vi "AMC Three Button Dialog.vi"(4 "Allow user to close window? (TRUE)":bool=TRUE, 5 "Justify Message (Left)":enum16{"Left", "Center", "Right"}(ring), 6 "Keyboard Shortcuts (Left is <Enter>)":T2={"Left Button Key Shortcut"={"Control"=FALSE, "Shift"=FALSE, "Key"="<Enter>"}, "Center Button Key Shortcut"={"Control"=FALSE, "Shift"=FALSE, "Key"=""}, "Right Button Key Shortcut"={"Control"=FALSE, "Shift"=FALSE, "Key"=""}}, 7 "Window Title (\"\")":string, 8 "Right Button Text (\"Cancel\")":string="Cancel", 9 "Center Button Text (\"No\")":string="No", 10 "Left Button Text (\"Yes\")":string="Yes", 11 "message":string) -> (3 "Which Button?":T3(ring)=enum."Center Button")   [LabVIEW 2009]
doc: "Displays text in a dialog with three buttons. The output enum indicates which of the three buttons the user chose, or it indicates that the user closed the dialog without making any choice."
uses:
  vi.lib/NI/AMC/AMC.lvlib
panel:
  in  "State Variables":T1={"Justify Message"=enum."Left", "message"="", "Left Button Text"="Yes", "Center Button Text"="No", "Right Button Text"="Cancel", "Keyboard Shortcuts"={"Left Button Key Shortcut"={"Control"=FALSE, "Shift"=FALSE, "Key"="<Enter>"}, "Center Button Key Shortcut"={"Control"=FALSE, "Shift"=FALSE, "Key"=""}, "Right Button Key Shortcut"={"Control"=FALSE, "Shift"=FALSE, "Key"=""}}, "Left Button Visible"=FALSE, "Center Button Visible"=FALSE, "Right Button Visible"=FALSE, "Minimum window width for buttons"=0, "Mimimum window width"=0, "Minimum width for message"=0, "FP Spacing"=12, "Height"=0, "Actual Width"=0, "Left Edge"=0, "FP Window Title"=""}
  in  "OK":string="OK"
  out "C-Message":string
  in  "Right Button":bool
  in  "Center Button":bool
  in  "Left Button":bool
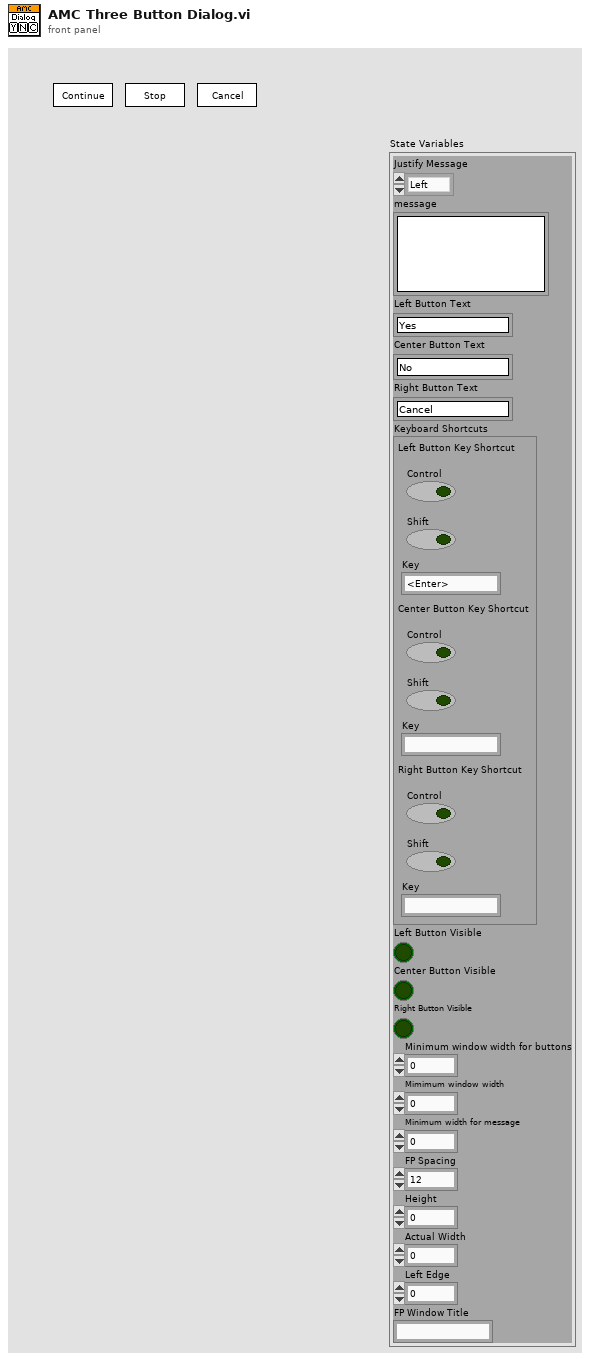
[diagram p1: front panel]
types:
  T1 = cluster{"Justify Message":enum16{"Left", "Center", "Right"}, "message":string, "Left Button Text":string, "Center Button Text":string, "Right Button Text":string, "Keyboard Shortcuts":cluster{"Left Button Key Shortcut":cluster{"Control":bool, "Shift":bool, "Key":string}, "Center Button Key Shortcut":cluster{"Control":bool, "Shift":bool, "Key":string}, "Right Button Key Shortcut":cluster{"Control":bool, "Shift":bool, "Key":string}}, "Left Button Visible":bool, "Center Button Visible":bool, "Right Button Visible":bool, "Minimum window width for buttons":i32, "Mimimum window width":i32, "Minimum width for message":i32, "FP Spacing":i32, "Height":u32, "Actual Width":i32, "Left Edge":i32, "FP Window Title":string}
  T2 = cluster{"Left Button Key Shortcut":cluster{"Control":bool, "Shift":bool, "Key":string}, "Center Button Key Shortcut":cluster{"Control":bool, "Shift":bool, "Key":string}, "Right Button Key Shortcut":cluster{"Control":bool, "Shift":bool, "Key":string}}
  T3 = enum16{"Left Button", "Center Button", "Right Button", "Window Close"}
  T4 = typedef "AMC.lvlib/Message Queue.ctl" = refnum<queue>
  T5 = cluster{"left":i16, "top":i16, "right":i16, "bottom":i16}
  T6 = cluster{"Control":bool, "Shift":bool, "Key":string}
  T7 = cluster{bool, "Control":bool, "Shift":bool, "Key":string}
  T8 = typedef "LVRectTypeDef.ctl" = cluster{"left":i16, "top":i16, "right":i16, "bottom":i16}
  T9 = typedef "LVPointTypeDef.ctl" = cluster{"Horizontal":i16, "Vertical":i16}
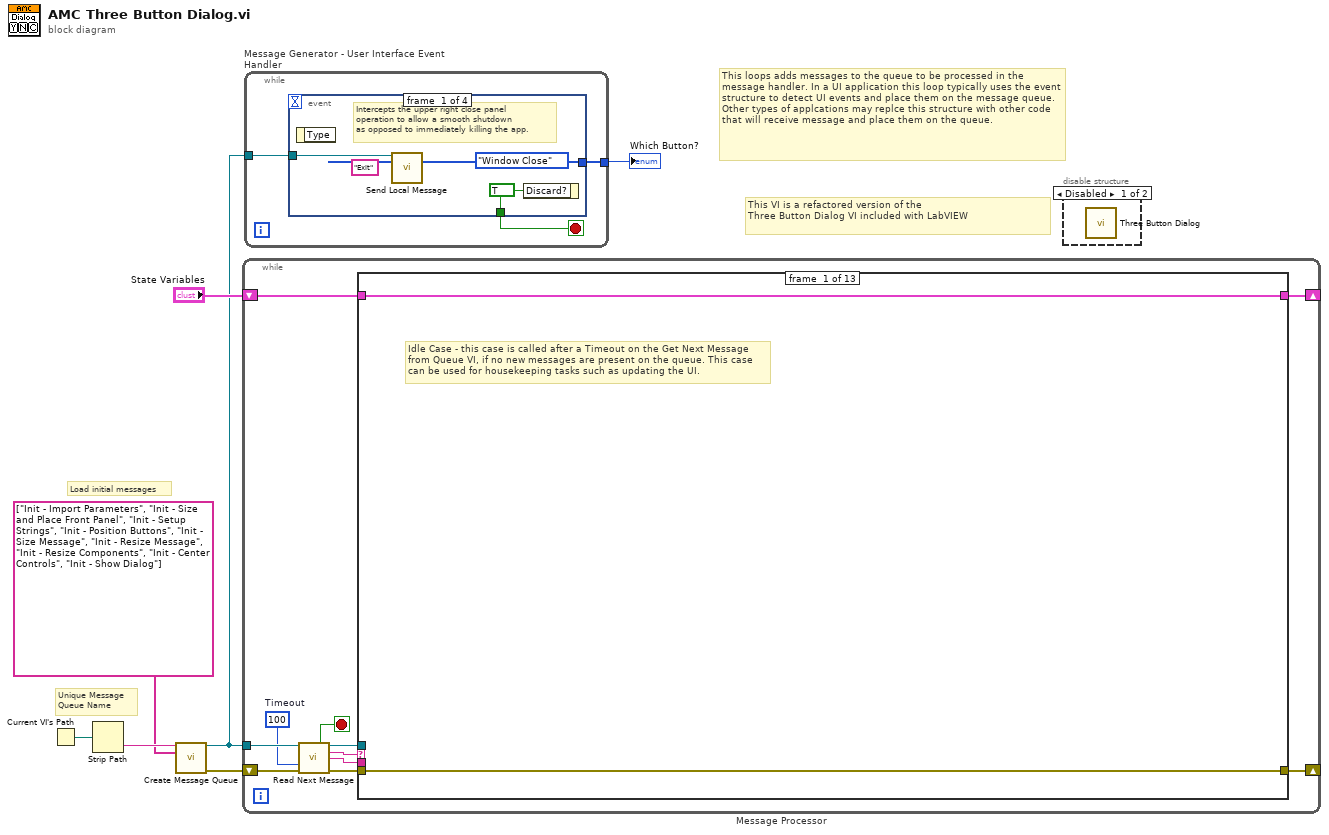
[diagram p0: block diagram]
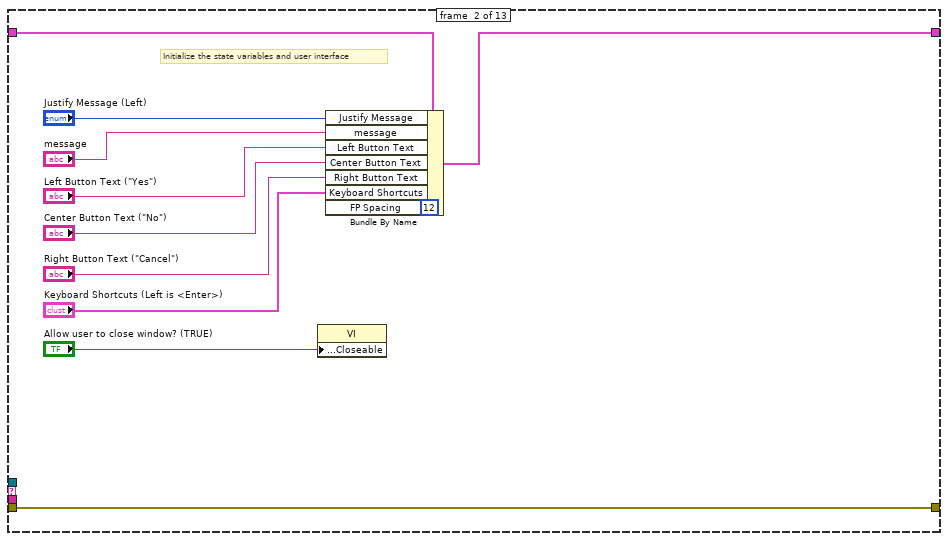
[diagram p3: hidden frame]
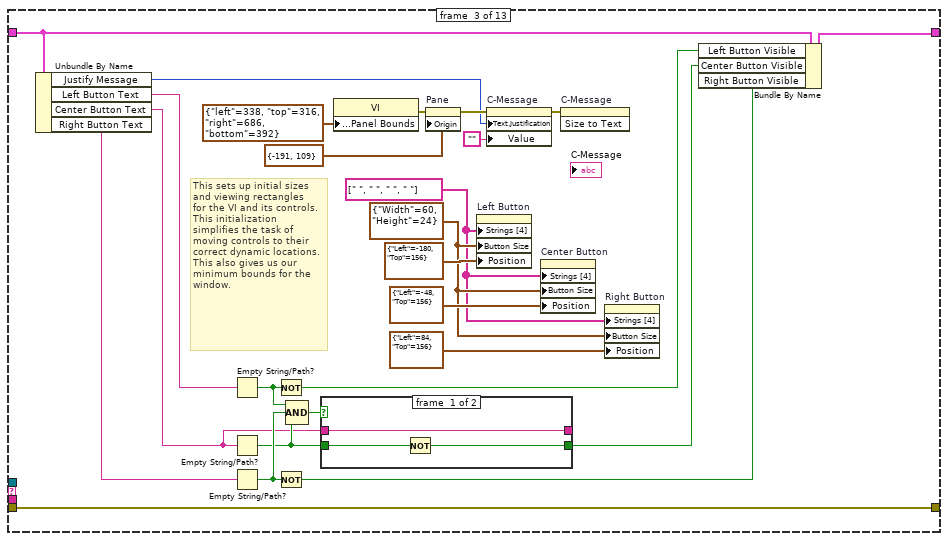
[diagram p4: hidden frame]
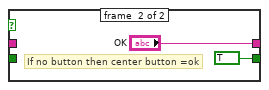
[diagram p5: hidden frame]
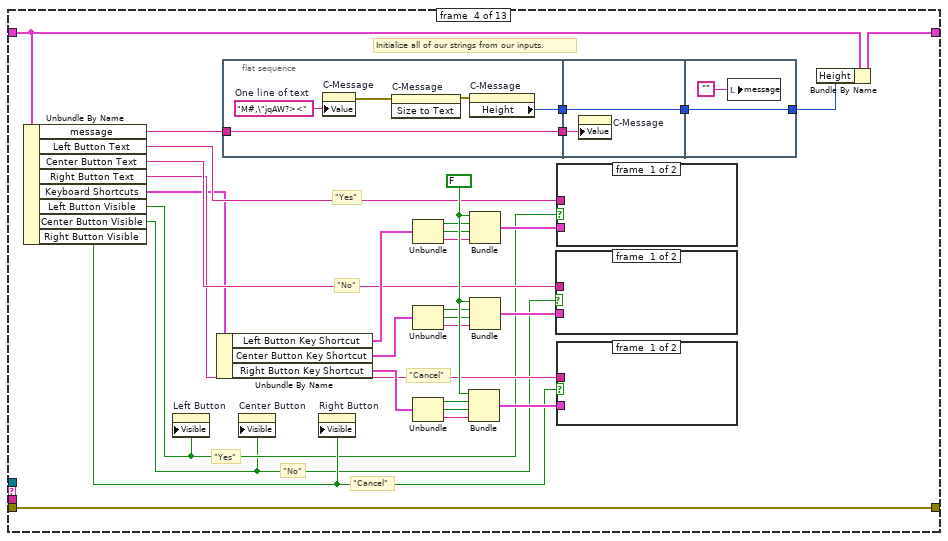
[diagram p6: hidden frame]
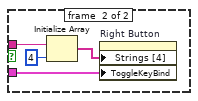
[diagram p7: hidden frame]
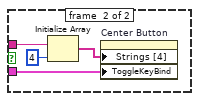
[diagram p8: hidden frame]
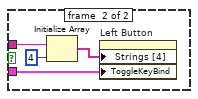
[diagram p9: hidden frame]
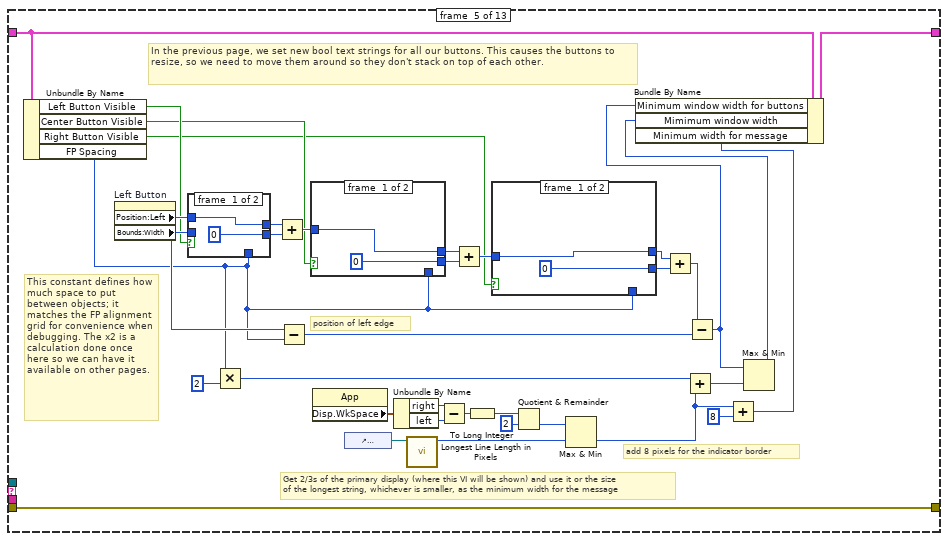
[diagram p10: hidden frame]
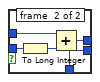
[diagram p11: hidden frame]
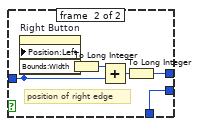
[diagram p12: hidden frame]
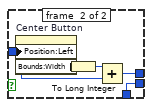
[diagram p13: hidden frame]
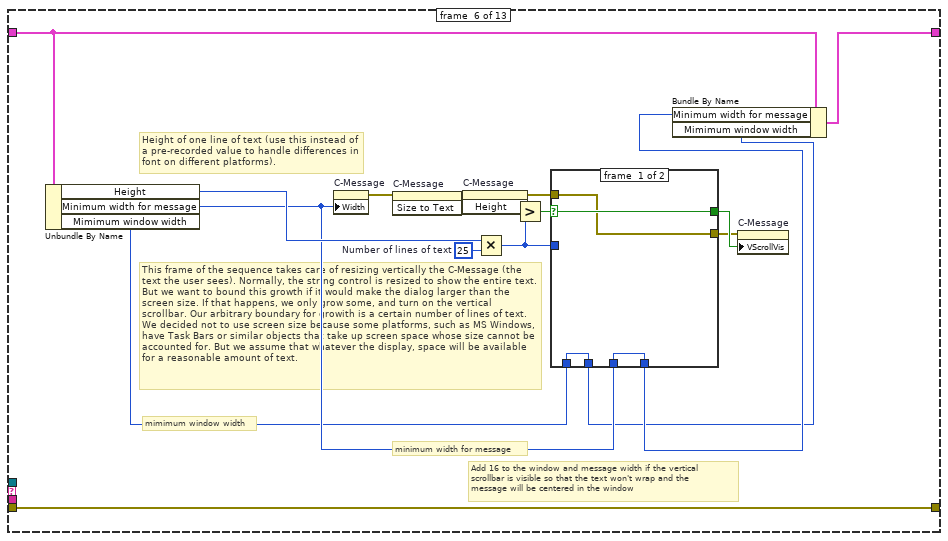
[diagram p14: hidden frame]
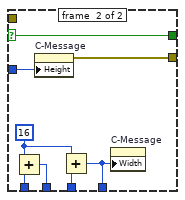
[diagram p15: hidden frame]
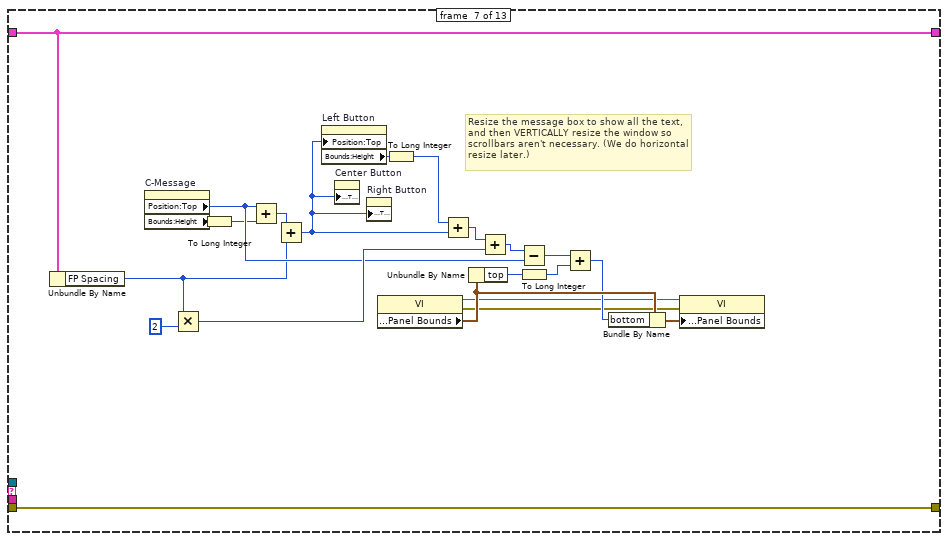
[diagram p16: hidden frame]
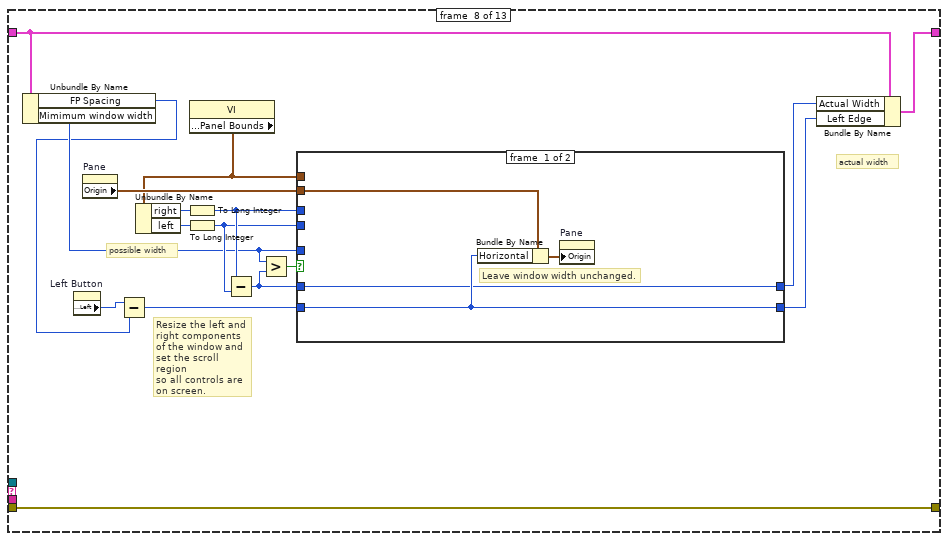
[diagram p17: hidden frame]
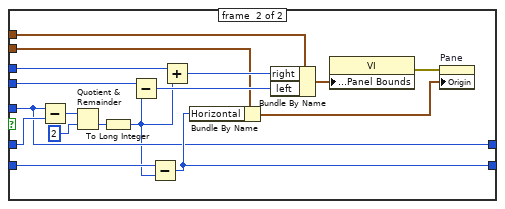
[diagram p18: hidden frame]
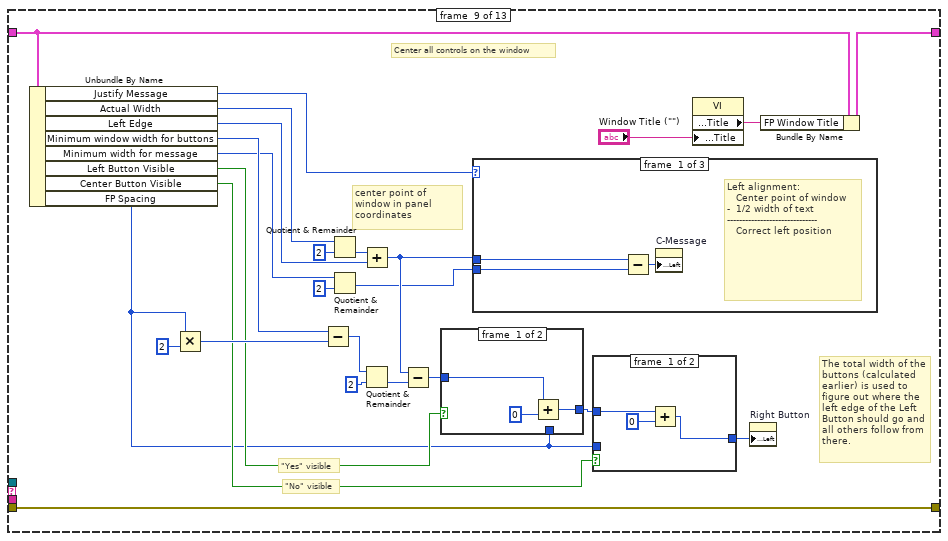
[diagram p19: hidden frame]
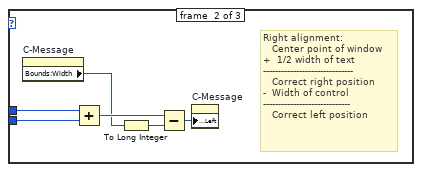
[diagram p20: hidden frame]
diagram:
  # "This VI is a refactored version of the\nThree Button Dialog VI included\twith LabVIEW"
  # "This loops adds messages to the queue to be processed in the message handler. In a UI application this loop typically uses the event structure to detect UI events and place them on the message queue. Other types of applcations may replce this structure with other code that will receive message and place them on the queue."
  # "Unique Message\nQueue Name"
  # "Load initial messages"
  n1 = Current VI's Path() -> (path=w6:path)
  n2 = Strip Path(path=w6) -> (name=w7:string)  [unwired: 1 out]
  n3 = call "Create Message Queue.vi"("message queue name"=w7, "initial message names"=string[] ["Init - Import Parameters", "Init - Size and Place Front Panel", "Init - Setup Strings", "Init - Position Buttons", "Init - Size Message", "Init - Resize Message", "Init - Resize Components", "Init - Center Controls", "Init - Show Dialog"]) -> ("message queue out"=w4:T4, "error out"=w3:errorcluster)  [unwired: 12 in]
  n4 = while "Message Processor" {
    shift-left: w3 -> [w12]
    shift-right: [w13] -> _
    tunnel: w4 -> [w11]
    shift-left: "State Variables" -> [w18]
    shift-right: [w17] -> _
    stop <- w16 stop-if-true
    w8 = 100  # Timeout
    n5 = call "Read Next Message.vi"("message queue in"=w11, "timeout (1 ms)"=w8, "error in"=w12) -> ("exit process?"=w16:bool, "message queue out"=w15:T4, "message name"=w10:string, "message value"=w9:string, "error out"=w14:errorcluster)  [unwired: 5 in, 3 out]
    n6 = case shown="\"Error\"" w10 {
      selector: w10 -> [_ _ _ _ _ _ _ _ _ _ _ _ w343]
      tunnel: [w20 w30 w37 w64 w149 w175 w203 w225 w283 w321 w334 w336 w345] -> w17
      tunnel: w18 -> [w20 w31 w38 w65 w122 w176 w203 w229 w285 w321 w334 w336 w345]
      tunnel: w15 -> [_ _ _ _ _ _ _ _ _ _ w332 w339 _]
      tunnel: w14 -> [w19 w22 w32 w62 w114 w172 w201 w224 w262 w323 _ w340 w344]
      tunnel: [w19 w22 w32 w62 w114 w172 w201 w224 w262 w323 errorcluster {"status"=FALSE, "code"=0, "source"=""} ("error out") w338 w344] -> w13
      tunnel: w9 -> [_ _ _ _ _ _ _ _ _ _ _ _ _]
      frame #0 {
        # "Idle Case - this case is called after a Timeout on the Get Next Message from Queue VI, if no new messages are present on the queue. This case can be used for housekeeping tasks such as updating the UI."
      }
      frame #1 {
        # "Initialize the state variables and user interface"
        n7 = property class="VI"("Front Panel Window:Closeable"="Allow user to close window? (TRUE)") -> ()  [unwired: 2 in, 2 out]
        n8 = Bundle By Name(cluster=w31, "Justify Message"="Justify Message (Left)", "message"="message", "Left Button Text"="Left Button Text (\"Yes\")", "Center Button Text"="Center Button Text (\"No\")", "Right Button Text"="Right Button Text (\"Cancel\")", "Keyboard Shortcuts"="Keyboard Shortcuts (Left is <Enter>)", "FP Spacing"=12) -> (w30:T1)
      }
      frame #2 {
        w46 = string[] [" ", " ", " ", " "] ("Strings [4]")
        w47 = cluster{"Width":u32, "Height":u32} {"Width"=60, "Height"=24} ("Button Size")
        # "This sets up initial sizes and viewing rectangles\nfor the VI and its controls. This initialization\nsimplifies the task of moving controls to their\ncorrect dynamic locations. This also gives us our\nminimum bounds for the window."
        n9 = Unbundle By Name(w38) -> ("Justify Message"=w36:enum16{"Left", "Center", "Right"}, "Left Button Text"=w39:string, "Center Button Text"=w40:string, "Right Button Text"=w41:string)
        n10 = Empty String/Path?(string/path=w39) -> (empty?=w42:bool)
        n11 = Empty String/Path?(string/path=w40) -> (empty?=w44:bool)
        n12 = Empty String/Path?(string/path=w41) -> (empty?=w45:bool)
        n13 = Not(x=w42) -> (.not. x?=w33:bool)
        n14 = Not(x=w45) -> (.not. x?=w35:bool)
        n15 = Compound Arithmetic op=AND(w42, w45, w44) -> (w43:bool)
        n16 = case shown="True" w43 {
          tunnel: w44 -> [w59 _]
          tunnel: [w58 TRUE] -> w34
          tunnel: w40 -> [w57 _]
          tunnel: [w57 "OK"] -> _
          frame #0 {
            n17 = Not(x=w59) -> (.not. x?=w58:bool)
          }
          frame #1 {
            # "If no button then center button =ok"
          }
        }
        n18 = property class="VI"("Front Panel Window:Panel Bounds"=T5 {"left"=338, "top"=316, "right"=686, "bottom"=392} ("Front Panel.PanelBounds")) -> (error out=w54:errorcluster)  [unwired: 2 in, 1 out]
        n19 = property on="Pane" class="Pane"(error in=w54, "Origin"=cluster{"Horizontal":i16, "Vertical":i16} {"Horizontal"=-191, "Vertical"=109} ("Front Panel.Origin")) -> (error out=w55:errorcluster)  [unwired: 1 in, 1 out]
        n20 = property on="Left Button" class="Boolean"("Strings [4]"=w46, "Button Size"=w47, "Position"=cluster{"Left":i32, "Top":i32} {"Left"=-180, "Top"=156}) -> ()  [unwired: 2 in, 2 out]
        n21 = property on="C-Message" class="Str"(error in=w55, "Text.Justification"=w36, "Value"="") -> (error out=w51:errorcluster)  [unwired: 1 in, 1 out]
        n22 = property on="Center Button" class="Bool"("Strings [4]"=w46, "Button Size"=w47, "Position"=cluster{"Left":i32, "Top":i32} {"Left"=-48, "Top"=156}) -> ()  [unwired: 2 in, 2 out]
        n23 = invoke on="C-Message" class="Str" method="Size to Text"(error in=w51) -> ()  [unwired: 2 in, 3 out]
        n24 = property on="Right Button" class="Bool"("Strings [4]"=w46, "Button Size"=w47, "Position"=cluster{"Left":i32, "Top":i32} {"Left"=84, "Top"=156}) -> ()  [unwired: 2 in, 2 out]
        n25 = Bundle By Name(cluster=w38, "Left Button Visible"=w33, "Center Button Visible"=w34, "Right Button Visible"=w35) -> (w37:T1)
      }
      frame #3 {
        w86 = FALSE
        # "\"Cancel\""
        # "\"No\""
        # "\"Yes\""
        # "\"Cancel\""
        # "\"No\""
        # "\"Yes\""
        # "Initialize all of our strings from our inputs."
        n26 = Unbundle By Name(w65) -> ("message"=w89:string, "Left Button Text"=w72:string, "Center Button Text"=w71:string, "Right Button Text"=w70:string, "Keyboard Shortcuts"=w69:T2, "Left Button Visible"=w67:bool, "Center Button Visible"=w66:bool, "Right Button Visible"=w68:bool)
        n27 = property on="Left Button" class="Boolean"("Visible"=w67) -> ()  [unwired: 2 in, 2 out]
        n28 = Unbundle By Name(w69) -> ("Left Button Key Shortcut"=w73:T6, "Center Button Key Shortcut"=w81:T6, "Right Button Key Shortcut"=w87:T6)
        n29 = flat-sequence {
          tunnel: [w106] -> w92
          tunnel: w89 -> [w105]
          tunnel: [w105] -> w91
          tunnel: w92 -> [w111]
          tunnel: [w111] -> w90
          tunnel: w91 -> [w110]
          tunnel: w90 -> [w112]
          tunnel: [w112] -> w63
          frame #0 {
            w109 = "M#,\"jqAW?><"  # One line of text
            n30 = property on="C-Message" class="Str"("Value"=w109) -> (error out=w107:errorcluster)  [unwired: 2 in, 1 out]
            n31 = invoke on="C-Message" class="Str" method="Size to Text"(error in=w107) -> (error out=w108:errorcluster)  [unwired: 2 in, 2 out]
            n32 = property on="C-Message" class="Str"(error in=w108) -> ("Height"=w106:u32)  [unwired: 1 in, 2 out]
          }
          frame #1 {
            n33 = property on="C-Message" class="Str"("Value"=w110) -> ()  [unwired: 2 in, 2 out]
          }
          frame #2 {
            n34 = local write "message"("") -> ()
          }
        }
        n35 = property on="Center Button" class="Bool"("Visible"=w66) -> ()  [unwired: 2 in, 2 out]
        n36 = property on="Right Button" class="Bool"("Visible"=w68) -> ()  [unwired: 2 in, 2 out]
        n37 = Unbundle(w73) -> ("Control"=w74:bool, "Shift"=w75:bool, "Key"=w76:string)
        n38 = Unbundle(w81) -> ("Control"=w78:bool, "Shift"=w79:bool, "Key"=w80:string)
        n39 = Unbundle(w87) -> ("Control"=w83:bool, "Shift"=w84:bool, "Key"=w85:string)
        n40 = Bundle(w86, "Control"=w83, "Shift"=w84, "Key"=w85) -> (w88:T7)  [unwired: 1 out]
        n41 = Bundle(w86, "Control"=w74, "Shift"=w75, "Key"=w76) -> (w77:T7)  [unwired: 1 out]
        n42 = Bundle(w86, "Control"=w78, "Shift"=w79, "Key"=w80) -> (w82:T7)  [unwired: 1 out]
        n43 = case shown="True" w66 {
          tunnel: w82 -> [_ w98]
          tunnel: w71 -> [_ w97]
          frame #0 {
          }
          frame #1 {
            n44 = Initialize Array(w97, 4 ("dimension size")) -> (w100:string[])
            n45 = property on="Center Button" class="Bool"("Strings [4]"=w100, "ToggleKeyBind"=w98) -> ()  [unwired: 2 in, 2 out]
          }
        }
        n46 = case shown="True" w67 {
          tunnel: w72 -> [_ w102]
          tunnel: w77 -> [_ w101]
          frame #0 {
          }
          frame #1 {
            n47 = Initialize Array(w102, 4 ("dimension size")) -> (w104:string[])
            n48 = property on="Left Button" class="Boolean"("Strings [4]"=w104, "ToggleKeyBind"=w101) -> ()  [unwired: 2 in, 2 out]
          }
        }
        n49 = case shown="True" w68 {
          tunnel: w88 -> [_ w94]
          tunnel: w70 -> [_ w93]
          frame #0 {
          }
          frame #1 {
            n50 = Initialize Array(w93, 4 ("dimension size")) -> (w96:string[])
            n51 = property on="Right Button" class="Bool"("Strings [4]"=w96, "ToggleKeyBind"=w94) -> ()  [unwired: 2 in, 2 out]
          }
        }
        n52 = Bundle By Name(cluster=w65, "Height"=w63) -> (w64:T1)
      }
      frame #4 {
        # "add 8 pixels for the indicator border"
        # "Get 2/3s of the primary display (where this VI will be shown) and use it or the size\nof the longest string, whichever is smaller, as the minimum width for the message"
        # "This constant defines how much space to put between objects; it matches the FP alignment grid for convenience when debugging. The x2 is a calculation done once here so we can have it available on other pages."
        # "In the previous page, we set new bool text strings for all our buttons. This causes the buttons to resize, so we need to move them around so they don't stack on top of each other."
        # "position of left edge"
        n53 = Unbundle By Name(w122) -> ("Left Button Visible"=w121:bool, "Center Button Visible"=w120:bool, "Right Button Visible"=w119:bool, "FP Spacing"=w118:i32)
        n54 = property on="Left Button" class="Boolean"() -> ("Position:Left"=w126:i32, "Bounds:Width"=w129:u32)  [unwired: 2 in, 2 out]
        n55 = case shown="True" w121 {
          tunnel: w126 -> [w151 w156]
          tunnel: w129 -> [_ w155]
          tunnel: [w151 w154] -> w132
          tunnel: w118 -> [_ w152]
          tunnel: [0 w152] -> w133
          frame #0 {
          }
          frame #1 {
            n56 = To Long Integer(number=w155) -> (32bit integer=w153:i32)
            n57 = Add(x=w156, y=w153) -> (x+y=w154:i32)
          }
        }
        n58 = Multiply(x=w118, y=2) -> (x*y=w138:i32)
        n59 = Add(x=w132, y=w133) -> (x+y=w128:i32)
        n60 = Subtract(x=w126, y=w118) -> (x-y=w125:i32)
        n61 = case shown="True" w120 {
          tunnel: w128 -> [w166 w171]
          tunnel: [w166 w170] -> w130
          tunnel: [0 w167] -> w134
          tunnel: w118 -> [_ w167]
          frame #0 {
          }
          frame #1 {
            n62 = property on="Center Button" class="Bool"("Position:Left"=w171) -> ("Bounds:Width"=w169:u32)  [unwired: 2 in, 2 out]
            n63 = To Long Integer(number=w169) -> (32bit integer=w168:i32)
            n64 = Add(x=w168, y=w171) -> (x+y=w170:i32)
          }
        }
        n65 = property class="App"() -> ("Disp.WkSpace"=w139:T8)  [unwired: 2 in, 2 out]
        n66 = control-ref of="C-Message"() -> (w136:refnum<vi>)
        n67 = Unbundle By Name(w139) -> ("right"=w143:i16, "left"=w144:i16)
        n68 = call <vilib>:"Longest Line Length in Pixels.vi"("String"=w136) -> ("longest line length"=w142:i32)  [unwired: 1 in, 8 out]
        n69 = Subtract(x=w143, y=w144) -> (x-y=w140:i16)
        n70 = Add(x=w130, y=w134) -> (x+y=w127:i32)
        n71 = To Long Integer(number=w140) -> (32bit integer=w145:i32)
        n72 = case shown="True" w119 {
          tunnel: w127 -> [w158 w164]
          tunnel: [w158 w162] -> w131
          tunnel: [0 w159] -> w135
          tunnel: w118 -> [_ w159]
          frame #0 {
          }
          frame #1 {
            # "position of right edge"
            n73 = property on="Right Button" class="Bool"("Position:Left"=w164) -> ("Bounds:Width"=w161:u32)  [unwired: 2 in, 2 out]
            n74 = To Long Integer(number=w161) -> (32bit integer=w160:i32)
            n75 = Add(x=w160, y=w164) -> (x+y=w163:i32)
            n76 = To Long Integer(number=w163) -> (32bit integer=w162:i32)
          }
        }
        n77 = Quotient & Remainder(x=w145, y=2) -> (floor(x/y)=w148:i32)  [unwired: 1 out]
        n78 = Max & Min(x=w148, y=w142) -> (min(x,y)=w147:i32)  [unwired: 1 out]
        n79 = Add(x=w131, y=w135) -> (x+y=w124:i32)
        n80 = Add(x=w138, y=w147) -> (x+y=w123:i32)
        n81 = Subtract(x=w124, y=w125) -> (x-y=w117:i32)
        n82 = Add(x=w147, y=8 ("x")) -> (x+y=w116:i32)
        n83 = Max & Min(x=w117, y=w123) -> (max(x,y)=w115:i32)  [unwired: 1 out]
        n84 = Bundle By Name(cluster=w122, "Minimum window width for buttons"=w117, "Mimimum window width"=w115, "Minimum width for message"=w116) -> (w149:T1)
      }
      frame #5 {
        w186 = u32 25  # Number of lines of text
        # "Add 16 to the window and message width if the vertical\nscrollbar is visible so that the text won't wrap and the \nmessage will be centered in the window"
        # "mimimum window width"
        # "minimum width for message"
        # "Height of one line of text (use this instead of a pre-recorded value to handle differences in font on different platforms)."
        # "This frame of the sequence takes care of resizing vertically the C-Message (the text the user sees). Normally, the string control is resized to show the entire text. But we want to bound this growth if it would make the dialog larger than the screen size. If that happens, we only grow some, and turn on the vertical scrollbar. Our arbitrary boundary for growith is a certain number of lines of text. We decided not to use screen size because some platforms, such as MS Windows, have Task Bars or similar objects that take up screen space whose size cannot be accounted for. But we assume that whatever the display, space will be available for a reasonable amount of text."
        n85 = Unbundle By Name(w176) -> ("Height"=w179:u32, "Minimum width for message"=w178:i32, "Mimimum window width"=w177:i32)
        n86 = property on="C-Message" class="Str"("Width"=w178) -> (error out=w188:errorcluster)  [unwired: 2 in, 1 out]
        n87 = invoke on="C-Message" class="Str" method="Size to Text"(error in=w188) -> (error out=w180:errorcluster)  [unwired: 2 in, 2 out]
        n88 = property on="C-Message" class="Str"(error in=w180) -> (error out=w185:errorcluster, "Height"=w181:u32)  [unwired: 1 in, 1 out]
        n89 = Multiply(x=w179, y=w186) -> (x*y=w187:u32)
        n90 = Greater?(x=w181, y=w187) -> (0:w182:bool)
        n91 = case shown="True" w182 {
          selector: w182 -> [w192 w199]
          tunnel: [w191 w200] -> w183
          tunnel: [w192 w199] -> w184
          tunnel: w185 -> [w191 _]
          tunnel: w187 -> [_ w198]
          tunnel: [w190 w196] -> w173
          tunnel: w177 -> [w190 w197]
          tunnel: [w189 w193] -> w174
          tunnel: w178 -> [w189 w195]
          frame #0 {
          }
          frame #1 {
            w194 = 16 ("x")
            n92 = Add(x=w194, y=w197) -> (x+y=w196:i32)
            n93 = property on="C-Message" class="Str"("Height"=w198) -> (error out=w200:errorcluster)  [unwired: 2 in, 1 out]
            n94 = Add(x=w194, y=w195) -> (x+y=w193:i32)
            n95 = property on="C-Message" class="Str"("Width"=w193) -> ()  [unwired: 2 in, 2 out]
          }
        }
        n96 = Bundle By Name(cluster=w176, "Minimum width for message"=w174, "Mimimum window width"=w173) -> (w175:T1)
        n97 = property on="C-Message" class="Str"(error in=w183, "VScrollVis"=w184) -> ()  [unwired: 1 in, 2 out]
      }
      frame #6 {
        # "Resize the message box to show all the text, and then VERTICALLY resize the window so scrollbars aren't necessary. (We do horizontal resize later.)"
        n98 = Unbundle By Name(w203) -> ("FP Spacing"=w202:i32)
        n99 = property on="C-Message" class="Str"() -> ("Position:Top"=w217:i32, "Bounds:Height"=w218:u32)  [unwired: 2 in, 2 out]
        n100 = Multiply(x=w202, y=2) -> (x*y=w222:i32)
        n101 = To Long Integer(number=w218) -> (32bit integer=w212:i32)
        n102 = Add(x=w217, y=w212) -> (x+y=w220:i32)
        n103 = Add(x=w220, y=w202) -> (x+y=w219:i32)
        n104 = property on="Left Button" class="Boolean"("Position:Top"=w219) -> ("Bounds:Height"=w215:u32)  [unwired: 2 in, 2 out]
        n105 = property on="Center Button" class="Bool"("Position:Top"=w219) -> ()  [unwired: 2 in, 2 out]
        n106 = property on="Right Button" class="Bool"("Position:Top"=w219) -> ()  [unwired: 2 in, 2 out]
        n107 = property class="VI"() -> (reference out=w206:refnum<vi>, error out=w205:errorcluster, "Front Panel Window:Panel Bounds"=w214:T8)  [unwired: 2 in]
        n108 = To Long Integer(number=w215) -> (32bit integer=w216:i32)
        n109 = Add(x=w216, y=w219) -> (x+y=w211:i32)
        n110 = Unbundle By Name(w214) -> ("top"=w208:i16)
        n111 = Add(x=w211, y=w222) -> (x+y=w210:i32)
        n112 = Subtract(x=w210, y=w217) -> (x-y=w207:i32)
        n113 = To Long Integer(number=w208) -> (32bit integer=w213:i32)
        n114 = Add(x=w207, y=w213) -> (x+y=w209:i32)
        n115 = Bundle By Name(cluster=w214, "bottom"=w209) -> (w204:T8)
        n116 = property class="VI"(reference=w206, error in=w205, "Front Panel Window:Panel Bounds"=w204) -> ()  [unwired: 2 out]
      }
      frame #7 {
        # "Resize the left and\nright components\nof the window and\nset the scroll region\nso all controls are \non screen."
        # "actual width"
        # "possible width"
        n117 = Unbundle By Name(w229) -> ("FP Spacing"=w223:i32, "Mimimum window width"=w226:i32)
        n118 = property on="Left Button" class="Boolean"() -> ("Position:Left"=w239:i32)  [unwired: 2 in, 2 out]
        n119 = property on="Pane" class="Pane"() -> ("Origin"=w238:T9)  [unwired: 2 in, 2 out]
        n120 = Subtract(x=w239, y=w223) -> (x-y=w235:i32)
        n121 = property class="VI"() -> ("Front Panel Window:Panel Bounds"=w233:T8)  [unwired: 2 in, 2 out]
        n122 = Unbundle By Name(w233) -> ("right"=w231:i16, "left"=w232:i16)
        n123 = To Long Integer(number=w231) -> (32bit integer=w237:i32)
        n124 = To Long Integer(number=w232) -> (32bit integer=w236:i32)
        n125 = Subtract(x=w237, y=w236) -> (x-y=w230:i32)
        n126 = Greater?(x=w226, y=w230) -> (0:w234:bool)
        n127 = case shown="True" w234 {
          tunnel: w230 -> [w241 w260]
          tunnel: w226 -> [_ w247]
          tunnel: w237 -> [_ w255]
          tunnel: w236 -> [_ w256]
          tunnel: w233 -> [_ w257]
          tunnel: [w243 w249] -> w227
          tunnel: w238 -> [w242 w250]
          tunnel: w235 -> [w243 w248]
          tunnel: [w241 w247] -> w228
          frame #0 {
            # "Leave window width unchanged."
            n128 = Bundle By Name(cluster=w242, "Horizontal"=w243) -> (w240:T9)
            n129 = property on="Pane" class="Pane"("Origin"=w240) -> ()  [unwired: 2 in, 2 out]
          }
          frame #1 {
            n130 = Subtract(x=w247, y=w260) -> (x-y=w259:i32)
            n131 = Quotient & Remainder(x=w259, y=2) -> (floor(x/y)=w252:i32)  [unwired: 1 out]
            n132 = To Long Integer(number=w252) -> (32bit integer=w246:i32)
            n133 = Subtract(x=w256, y=w246) -> (x-y=w253:i32)
            n134 = Subtract(x=w248, y=w246) -> (x-y=w249:i32)
            n135 = Add(x=w255, y=w246) -> (x+y=w254:i32)
            n136 = Bundle By Name(cluster=w250, "Horizontal"=w249) -> (w244:T9)
            n137 = Bundle By Name(cluster=w257, "right"=w254, "left"=w253) -> (w251:T8)
            n138 = property class="VI"("Front Panel Window:Panel Bounds"=w251) -> (error out=w245:errorcluster)  [unwired: 2 in, 1 out]
            n139 = property on="Pane" class="Pane"(error in=w245, "Origin"=w244) -> ()  [unwired: 1 in, 2 out]
          }
        }
        n140 = Bundle By Name(cluster=w229, "Actual Width"=w228, "Left Edge"=w227) -> (w225:T1)
      }
      frame #8 {
        # "\"No\" visible"
        # "\"Yes\" visible"
        # "The total width of the buttons (calculated earlier) is used to figure out where the left edge of the Left Button should go and all others follow from there."
        # "center point of window in panel coordinates"
        # "Center all controls on the window"
        n141 = Unbundle By Name(w285) -> ("Justify Message"=w269:enum16{"Left", "Center", "Right"}, "Actual Width"=w268:i32, "Left Edge"=w267:i32, "Minimum window width for buttons"=w266:i32, "Minimum width for message"=w265:i32, "Left Button Visible"=w264:bool, "Center Button Visible"=w263:bool, "FP Spacing"=w261:i32)
        n142 = Multiply(x=w261, y=2) -> (x*y=w282:i32)
        n143 = Subtract(x=w266, y=w282) -> (x-y=w273:i32)
        n144 = Quotient & Remainder(x=w268, y=2) -> (floor(x/y)=w271:i32)  [unwired: 1 out]
        n145 = Quotient & Remainder(x=w265, y=2) -> (floor(x/y)=w279:i32)  [unwired: 1 out]
        n146 = Add(x=w271, y=w267) -> (x+y=w280:i32)
        n147 = Quotient & Remainder(x=w273, y=2) -> (floor(x/y)=w274:i32)  [unwired: 1 out]
        n148 = Subtract(x=w280, y=w274) -> (x-y=w275:i32)
        n149 = case shown="True" w264 {
          tunnel: w261 -> [_ w317]
          tunnel: w275 -> [w312 w316]
          tunnel: [w311 w314] -> w276
          frame #0 {
            n150 = Add(x=w312, y=0) -> (x+y=w311:i32)
          }
          frame #1 {
            n151 = property on="Left Button" class="Bool"("Position:Left"=w316) -> ("Bounds:Width"=w315:u32)  [unwired: 2 in, 2 out]
            n152 = To Long Integer(number=w315) -> (32bit integer=w313:i32)
            n153 = Compound Arithmetic op=ADD(w313, w316, w317) -> (w314:i32)
          }
        }
        n154 = case shown="\"Right\"" w269 {
          tunnel: w280 -> [w289 w295 w297]
          tunnel: w279 -> [w287 w294 _]
          frame #0 {
            # "Left alignment:\n   Center point of window\n-  1/2 width of text\n------------------------------\n   Correct left position"
            n155 = Subtract(x=w289, y=w287) -> (x-y=w288:i32)
            n156 = property on="C-Message" class="Str"("Position:Left"=w288) -> ()  [unwired: 2 in, 2 out]
          }
          frame #1 {
            # "Right alignment:\n   Center point of window\n+  1/2 width of text\n------------------------------\n   Correct right position\n-  Width of control\n-----------------------------\n   Correct left position"
            n157 = property on="C-Message" class="Str"() -> ("Bounds:Width"=w291:u32)  [unwired: 2 in, 2 out]
            n158 = Add(x=w295, y=w294) -> (x+y=w293:i32)
            n159 = To Long Integer(number=w291) -> (32bit integer=w290:i32)
            n160 = Subtract(x=w293, y=w290) -> (x-y=w292:i32)
            n161 = property on="C-Message" class="Str"("Position:Left"=w292) -> ()  [unwired: 2 in, 2 out]
          }
          frame #2 {
            # "Center alignment:\n   Center point of window\n-  1/2 width of control\n------------------------------\n   Correct left position\n\n(the text is itself centered in the control, so centering control centers text)"
            n162 = property on="C-Message" class="Str"() -> ("Bounds:Width"=w300:u32)  [unwired: 2 in, 2 out]
            n163 = To Long Integer(number=w300) -> (32bit integer=w298:i32)
            n164 = Quotient & Remainder(x=w298, y=2) -> (floor(x/y)=w296:i32)  [unwired: 1 out]
            n165 = Subtract(x=w297, y=w296) -> (x-y=w299:i32)
            n166 = property on="C-Message" class="Str"("Position:Left"=w299) -> ()  [unwired: 2 in, 2 out]
          }
        }
        n167 = case shown="True" w263 {
          tunnel: w261 -> [_ w309]
          tunnel: w276 -> [w304 w307]
          tunnel: [w303 w306] -> w277
          frame #0 {
            n168 = Add(x=w304, y=0) -> (x+y=w303:i32)
          }
          frame #1 {
            n169 = property on="Center Button" class="Bool"("Position:Left"=w307) -> ("Bounds:Width"=w308:u32)  [unwired: 2 in, 2 out]
            n170 = To Long Integer(number=w308) -> (32bit integer=w305:i32)
            n171 = Compound Arithmetic op=ADD(w305, w307, w309) -> (w306:i32)
          }
        }
        n172 = property class="VI"("Front Panel Window:Title"="Window Title (\"\")") -> ("Front Panel Window:Title"=w284:string)  [unwired: 2 in, 2 out]
        n173 = property on="Right Button" class="Bool"("Position:Left"=w277) -> ()  [unwired: 2 in, 2 out]
        n174 = Bundle By Name(cluster=w285, "FP Window Title"=w284) -> (w283:T1)
      }
      frame #9 {
        # "\"No\" visible"
        # "\"Yes\" visible"
        # "This code assigns key focus to\nthe left-most visible button."
        n175 = Unbundle By Name(w321) -> ("Left Button Visible"=w320:bool, "Center Button Visible"=w319:bool)
        n176 = invoke class="VI" method="FP.Center"() -> (error out=w322:errorcluster)  [unwired: 3 in, 2 out]
        n177 = property class="VI"(error in=w322, "Front Panel.Open"=TRUE ("Front Panel Window:Open")) -> (error out=w318:errorcluster)  [unwired: 1 in, 1 out]
        n178 = case shown="True" w320 {
          tunnel: w319 -> [w329 _]
          tunnel: w318 -> [_ _]
          frame #0 {
            n179 = control-ref of="Center Button"() -> (w328:refnum<vi>)
            n180 = control-ref of="Right Button"() -> (w327:refnum<vi>)
            n181 = Select(t=w328, s=w329, f=w327) -> (s? t:f=w326:refnum<vi>)
            n182 = property class="Bool"(reference=w326, "Key Focus"=TRUE) -> ()  [unwired: 1 in, 2 out]
          }
          frame #1 {
            n183 = property on="Left Button" class="Bool"("Key Focus"=TRUE) -> ()  [unwired: 2 in, 2 out]
          }
        }
      }
      frame #10 {
        # "Proceed to Exit - remove if this is\nnot appropriate for the General Error case"
        # "General Error Case - this case is called if an error is passed using the error cluster below. Typically most new errors should be handed in each individual case and not passed in the rror cluster. If necessary a custom error handler case should be added and called from other cases."
        n184 = call "Send Local Message.vi"("message queue in"=w332, "message name"="Exit") -> ()  [unwired: 11 in, 3 out]
      }
      frame #11 {
        # "Perform cleanup tasks.\nClear display before closing"
        n185 = call "Destroy Message Queue.vi"("message queue in"=w339, "error in"=w340) -> ("error out"=w338:errorcluster)  [unwired: 11 in, 2 out]
        n186 = Unbundle By Name(w336) -> ("FP Window Title"=w335:string)
        n187 = property class="VI"("Front Panel Window:Open"=FALSE, "Front Panel Window:Title"=w335) -> ()  [unwired: 2 in, 2 out]
      }
      frame #12 {
        # "Call this case if a message is received that is not handled \nby any other case. Typically this is a programming error\nas a result of a typo or unhandled message/missing message handler."
        n188 = Format Into String(format string="DevError: Missing message handler for '%s\" message." ("message"), w343) -> (resulting string=w341:string)  [unwired: 2 in, 1 out]
        n189 = One Button Dialog(message=w341) -> ()  [unwired: 2 out]
      }
    }
  }
  n190 = while "Message Generator - User Interface Event Handler" {
    tunnel: w4 -> [w347]
    tunnel: [w346] -> w2
    stop <- w348 stop-if-true
    n191 = event shown="[1] \"Left Button\": Value Change" {
      selector: _ -> [_ _ _ _]
      dyn-events: _ -> [_ _ _ _]
      timeout: _ -> [_ _ _ _]
      tunnel: [w352 TRUE ("Discard?") TRUE ("Discard?") TRUE ("Discard?")] -> w348
      tunnel: w347 -> [w351 w355 w359 w363]
      tunnel: [T3."Window Close" ("Which Button?") T3."Left Button" ("Which Button?") T3."Center Button" ("Which Button?") T3."Right Button" ("Which Button?")] -> w346
      event #0 {
        w352 = TRUE ("Discard?")
        # "Intercepts the upper right close panel\noperation to allow a smooth shutdown\nas opposed to immediately killing the app."
        n192 = event-data() -> ()  [unwired: 2 out]
        n193 = call "Send Local Message.vi"("message queue in"=w351, "message name"="Exit") -> ()  [unwired: 11 in, 3 out]
        n194 = event-data("Discard?"=w352) -> ()  [unwired: 1 in, 1 out]
      }
      event #1 {
        n195 = event-data() -> ()  [unwired: 2 out]
        n196 = call "Send Local Message.vi"("message queue in"=w355, "message name"="Exit") -> ()  [unwired: 11 in, 3 out]
      }
      event #2 {
        n197 = event-data() -> ()  [unwired: 2 out]
        n198 = call "Send Local Message.vi"("message queue in"=w359, "message name"="Exit") -> ()  [unwired: 11 in, 3 out]
      }
      event #3 {
        n199 = event-data() -> ()  [unwired: 2 out]
        n200 = call "Send Local Message.vi"("message queue in"=w363, "message name"="Exit") -> ()  [unwired: 11 in, 3 out]
      }
    }
  }
  "Which Button?" <- w2
  n201 = disable-structure shown="Disabled" {
    frame #0 {
      n202 = call <vilib>:"Three Button Dialog.vi"() -> ()  [unwired: 11 in, 1 out]
    }
    frame #1 {
    }
  }
